vi "BreadthSearch.vi"(6 "Path in":refnum<data-value>[](array[refnum]), 8 "error in (no error)":errorcluster, 10 "GraphNode in":refnum<data-value>, 11 "GraphSearch in":refnum<class "GraphSearch.lvclass">) -> (0 "error out":errorcluster, 1 "found":bool, 2 "GraphNode out":refnum<data-value>, 3 "GraphSearch out":refnum<class "GraphSearch.lvclass">, 4 "Path out":refnum<data-value>[](array[refnum]))   [LabVIEW 2009, in "GraphSearch.lvclass"]
uses:
  GraphSearch.lvclass
  GraphNode/GraphNode.lvclass
  Node/Node.lvclass
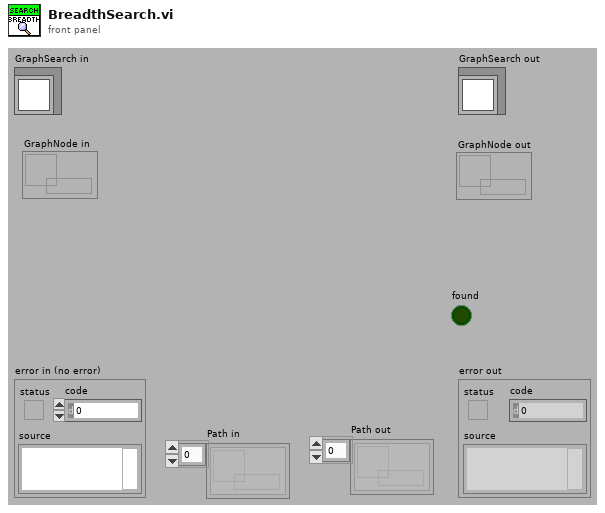
[diagram p1: front panel]
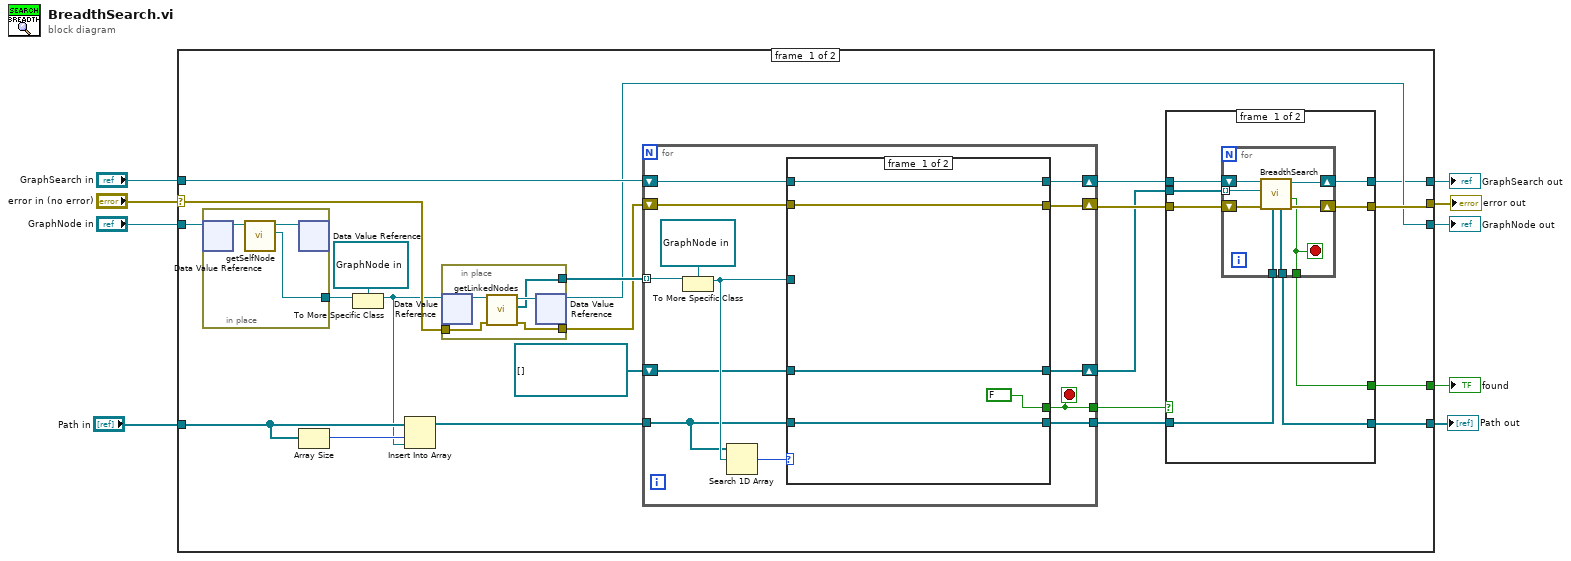
[diagram p0: block diagram]
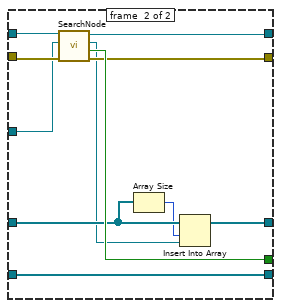
[diagram p3: hidden frame]
diagram:
  n1 = case shown="No Error" "error in (no error)" {
    selector: "error in (no error)" -> [w24 w92]
    tunnel: [w18 w92] -> w8
    tunnel: [w16 w91] -> w6
    tunnel: "GraphSearch in" -> [w25 w91]
    tunnel: "GraphNode in" -> [w31 w90]
    tunnel: "Path in" -> [w28 w89]
    tunnel: [w14 w89] -> w3
    tunnel: [w12 _] -> w2
    tunnel: [w17 w90] -> w1
    frame #0 {
      n2 = in-place {
        in-place-border: [w86] -> w30
        n3 = in-place-dvr #1(w31) -> (w88:refnum<class "GraphNode.lvclass">)  [unwired: 1 out]
        n4 = call "getSelfNode.vi"("Node in"=w88) -> ("selfNode"=w86:refnum<data-value>, "Node out"=w87:refnum<class "GraphNode.lvclass">)  [unwired: 8 in, 1 out]
        n5 = in-place-dvr #1(w87) -> ()  [unwired: 2 out]
      }
      n6 = Array Size(array=w28) -> (size(s)=w26:i32)
      n7 = To More Specific Class(target class=refnum<data-value> refnum ("GraphNode out"), reference=w30) -> (specific class reference=w21:refnum<data-value>)  [unwired: 1 in, 1 out]
      n8 = Insert Into Array(array=w28, index=w26, new element=w21) -> (w27:refnum<data-value>[])
      n9 = in-place {
        in-place-border: w24 -> [w83]
        in-place-border: [w82] -> w22
        in-place-border: [w81] -> w23
        n10 = in-place-dvr #2(w21) -> (w85:refnum<class "GraphNode.lvclass">)  [unwired: 1 out]
        n11 = call "getLinkedNodes.vi"("error in (no error)"=w83, "GraphNode in"=w85) -> ("error out"=w82:errorcluster, "LinkedNodes"=w81:refnum<data-value>[], "GraphNode out"=w84:refnum<class "GraphNode.lvclass">)  [unwired: 7 in]
        n12 = in-place-dvr #2(w84) -> (w17:refnum<data-value>)  [unwired: 1 out]
      }
      n13 = for {
        shift-right: [w63] -> w20
        shift-left: w25 -> [w64]
        tunnel: w23 -> [w62] mode=indexing
        tunnel: w27 -> [w57]
        tunnel: [w58] -> w13
        shift-right: [w55] -> w19
        shift-left: w22 -> [w56]
        tunnel: [w54] -> w15
        shift-right: [w52] -> w10
        shift-left: refnum<data-value>[] [] ("LinkedNodes") -> [w53]
        stop <- w58 stop-if-true
        n14 = To More Specific Class(target class=refnum<data-value> refnum ("GraphNode out"), reference=w62) -> (specific class reference=w59:refnum<data-value>)  [unwired: 1 in, 1 out]
        n15 = Search 1D Array(1D array=w57, element=w59) -> (index of element=w60:i32)  [unwired: 1 in]
        n16 = case shown="-1" w60 {
          tunnel: w64 -> [w69 w80]
          tunnel: [w69 w79] -> w63
          tunnel: w59 -> [_ w77]
          tunnel: [FALSE w75] -> w58
          tunnel: w57 -> [w66 w76]
          tunnel: w56 -> [w67 w78]
          tunnel: [w67 w74] -> w55
          tunnel: [w66 w76] -> w54
          tunnel: w53 -> [w65 w72]
          tunnel: [w65 w73] -> w52
          frame #0 {
          }
          frame #1 {
            n17 = call "SearchNode.vi"("error in (no error)"=w78, "GraphNode in"=w77, "GraphSearch in"=w80) -> ("error out"=w74:errorcluster, "found"=w75:bool, "GraphNode out"=w70:refnum<data-value>, "GraphSearch out"=w79:refnum<class "GraphSearch.lvclass">)  [unwired: 5 in]
            n18 = Array Size(array=w72) -> (size(s)=w71:i32)
            n19 = Insert Into Array(array=w72, index=w71, new element=w70) -> (w73:refnum<data-value>[])
          }
        }
      }
      n20 = case shown="False" w13 {
        selector: w13 -> [_ w48]
        tunnel: w20 -> [w39 w51]
        tunnel: w19 -> [w38 w50]
        tunnel: [w37 w50] -> w18
        tunnel: w10 -> [w36 _]
        tunnel: [w35 w51] -> w16
        tunnel: w15 -> [w34 w49]
        tunnel: [w33 w49] -> w14
        tunnel: [w32 w48] -> w12
        frame #0 {
          n21 = for {
            shift-right: [w46] -> w35
            shift-left: w39 -> [w47]
            shift-right: [w44] -> w37
            shift-left: w38 -> [w45]
            tunnel: w36 -> [w43] mode=indexing
            tunnel: w34 -> [w42]
            tunnel: [w41] -> w33
            tunnel: [w40] -> w32
            stop <- w40 stop-if-true
            n22 = call "BreadthSearch.vi"("Path in"=w42, "error in (no error)"=w45, "GraphNode in"=w43, "GraphSearch in"=w47) -> ("error out"=w44:errorcluster, "found"=w40:bool, "GraphSearch out"=w46:refnum<class "GraphSearch.lvclass">, "Path out"=w41:refnum<data-value>[])  [unwired: 3 in, 1 out]
          }
        }
        frame #1 {
        }
      }
    }
    frame #1 {
    }
  }
  "error out" <- w8
  "GraphSearch out" <- w6
  "Path out" <- w3
  "GraphNode out" <- w1
  "found" <- w2
